vi "QuadSubVINegativeMarcoGonzalez.vi"(1 "c":dbl, 2 "b":dbl, 3 "a":dbl) -> (0 "x2":dbl)   [LabVIEW 2012]
panel:
  # "Marco Gonzalez\nEA 3\n03 / 02 /2017"
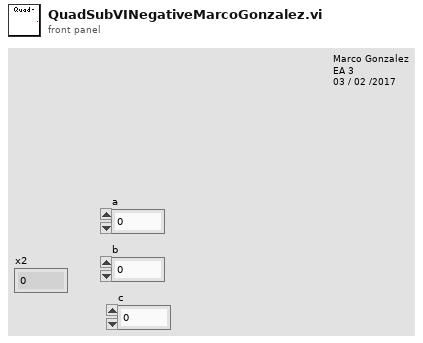
[diagram p1: front panel]
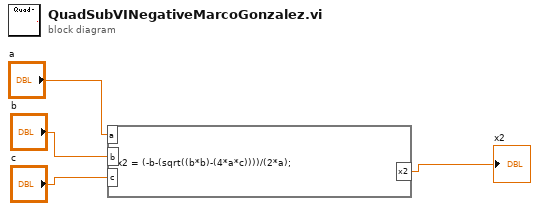
[diagram p0: block diagram]
diagram:
  n1 = formula code="x2 = (-b-(sqrt((b*b)-(4*a*c))))/(2*a);"("c"="c", "b"="b", "a"="a") -> ("x2"=→"x2":dbl)
